vi "I16toU16_poly.vi"   [LabVIEW 2010]
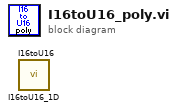
[diagram p0: block diagram]
diagram:
  n1 = call "I16toU16_1D.vi"() -> ()  [unwired: 1 in, 1 out]
  n2 = call "I16toU16.vi"() -> ()  [unwired: 1 in, 1 out]
